vi "labSSH_Commands.vi"(0 "Data":string, 1 "New_FGGA=T\nOld_FGGA=F":bool) -> (15 "error out":errorcluster)   [LabVIEW 2014]
uses:
  <vilib>/Labwerx/labSSH/labSSH.lvlib
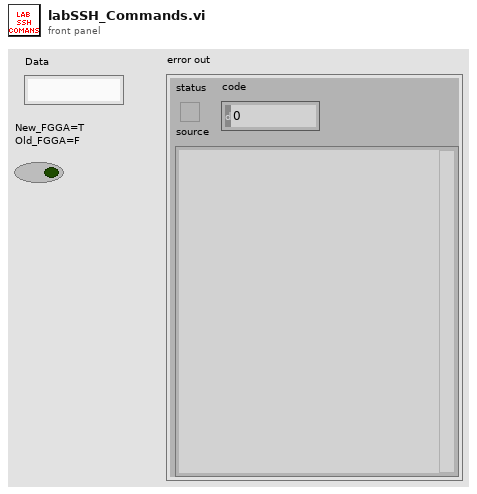
[diagram p1: front panel]
types:
  T1 = enum32{"Keyboard Interactive", "Password", "Public Key"}
  T2 = enum32{"invalid app kind", "Development System", "Run Time System", "Student Edition", "Embedded LabVIEW", "Evaluation", "Custom"}
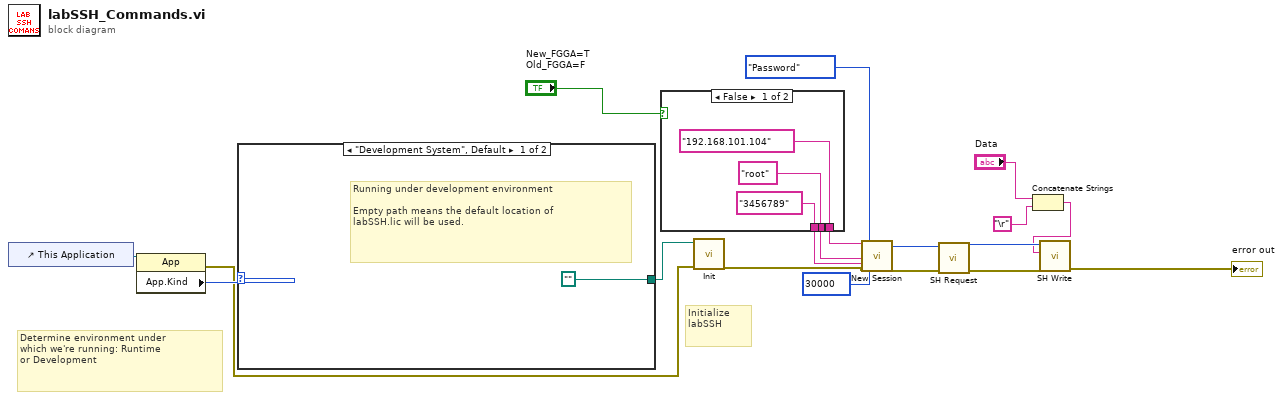
[diagram p0: block diagram]
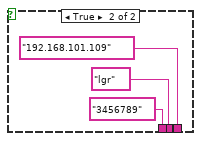
[diagram p2: hidden frame]
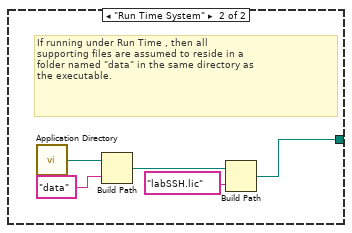
[diagram p3: hidden frame]
diagram:
  # "Initialize \nlabSSH"
  # "Determine environment under\nwhich we're running: Runtime\nor Development"
  n1 = control-ref of="This Application"() -> (w6:refnum<vi>)
  n2 = property class="App"(reference=w6) -> (error out=w3:errorcluster, "App.Kind"=w5:T2)  [unwired: 1 in, 1 out]
  n3 = case shown="\"Development System\", Default" w5 {
    tunnel: [path "" w22] -> w4
    frame "Development System", Default {
      # "Running under development environment\n\nEmpty path means the default location of\nlabSSH.lic will be used."
    }
    frame "Run Time System" {
      # "If running under Run Time , then all\nsupporting files are assumed to reside in a \nfolder named \"data\" in the same directory as\nthe executable."
      n4 = call <vilib>:"Application Directory.vi"() -> ("Application Directory"=w21:path)
      n5 = Build Path(base path=w21, name or relative path="data") -> (appended path=w23:path)
      n6 = Build Path(base path=w23, name or relative path="labSSH.lic") -> (appended path=w22:path)
    }
  }
  n7 = case shown="False" "New_FGGA=T\nOld_FGGA=F" {
    tunnel: ["192.168.101.104" ("IP Addr or Hostname") "192.168.101.109" ("IP Addr or Hostname")] -> w18
    tunnel: ["root" ("Username") "lgr" ("Username")] -> w17
    tunnel: ["3456789" ("Password") "3456789" ("Password")] -> w16
    frame False {
    }
    frame True {
    }
  }
  n8 = call <vilib>:"Init.vi"("error in (no error)"=w3, "License File Path Override"=w4) -> ("error out"=w19:errorcluster)  [unwired: 9 in]
  n9 = call <vilib>:"New Session.vi"("IP Addr or Hostname"=w18, "Username"=w17, "Password"=w16, "error in (no error)"=w19, "Authentication Type (Password)"=T1."Password", "Timeout msec (10000)"=30000) -> ("New LabSSH Session"=w15:u64, "error out"=w14:errorcluster)  [unwired: 12 in]
  n10 = call <vilib>:"SH Request.vi"("error in (no error)"=w14, "LabSSH Session"=w15) -> ("error out"=w13:errorcluster, "LabSSH Session Out"=w12:u64)  [unwired: 8 in]
  n11 = Concatenate Strings("Data", "\r") -> (w8:string)
  n12 = call <vilib>:"SH Write.vi"("error in (no error)"=w13, "Data"=w8, "LabSSH Session"=w12) -> ("error out"=→"error out":errorcluster)  [unwired: 6 in, 2 out]
